vi "SLSC_Check Connection and Module.vi"(8 "error in (no error)":errorcluster, 10 "compiled.settings":T3={"Name"="", "SLSC IP -Module Name"="", "Slot #"=0, "Configuration Data"={"Properties"={"Boolean Properties"=[], "Double Properties"=[], "I32 Properties"=[], "I64 Properties"=[], "String Properties"=[], "U32 Properties"=[], "U64 Properties"=[]}}, "SLSC Set Properties"=[], "SLSC Get Properties"=[], "SLSC Commands"=[], "Username"="admin", "Password"="", "Support Modules"=[]} {"Configuration Data"."Properties"."U64 Properties"."UInt64 Write" format="%.0x"; "Configuration Data"."Properties"."U32 Properties"."UInt32 Write" format="%.0x"; "Configuration Data"."Properties"."Double Properties"."Double Write" format="%_20g"}, 11 "Item Ref in":T2 format="%.0x") -> (0 "error out":errorcluster, 1 "Device Found?":bool, 2 "compiled.settings out":T3={"Name"="", "SLSC IP -Module Name"="", "Slot #"=0, "Configuration Data"={"Properties"={"Boolean Properties"=[], "Double Properties"=[], "I32 Properties"=[], "I64 Properties"=[], "String Properties"=[], "U32 Properties"=[], "U64 Properties"=[]}}, "SLSC Set Properties"=[], "SLSC Get Properties"=[], "SLSC Commands"=[], "Username"="admin", "Password"="", "Support Modules"=[]} {"Configuration Data"."Properties"."U64 Properties"."UInt64 Write" format="%.0x"; "Configuration Data"."Properties"."U32 Properties"."UInt32 Write" format="%.0x"; "Configuration Data"."Properties"."Double Properties"."Double Write" format="%_20g"}, 3 "Item Ref out":T2 format="%.0x")   [LabVIEW 2020, in "SLSC-12201 DIO Engine.lvlib"]
uses:
  SLSC-12201 DIO Engine.lvlib
  Shared/Compiled.Settings
  Shared/SLSC Dynamic Channel.ctl
  Shared/SLSC Dynamic Channel Type.ctl
  <vilib>/NI VeriStand/Custom Device API/Custom Device Item Ref.ctl
  <vilib>/NI VeriStand/Custom Device Tools/Custom Device Utility Library/RT Debug String Color Spec.ctl
  <vilib>/SLSC/Initialize Session with Devices.vi
  <vilib>/SLSC/Close Session.vi
  <vilib>/SLSC/SLSC.lvlib
  <resource>/objmgr/slsc.rc
  <vilib>/SLSC/Initialize Session without Resources.vi
  <vilib>/NI VeriStand/Custom Device Tools/Custom Device Utility Library/Custom Device Utility Library.lvlib
  Shared/SLSC-12201 DIO Shared.lvlib
  <vilib>/NI VeriStand/Custom Device API/Custom Device API.lvlib
panel:
  out "Supported Modules":T1(array[cluster]) {"Dev.ProductNumber" format="%.0x"; "Dev.VendorNumber" format="%.0x"}
  out "Dev.VendorNum":u32 format="%.0x"
  out "Dev.ProductNum":u32 format="%.0x"
  out "Dev.ProductName":string
  in  "Connect timeout (s)":dbl=20.0 format="%#_13g"
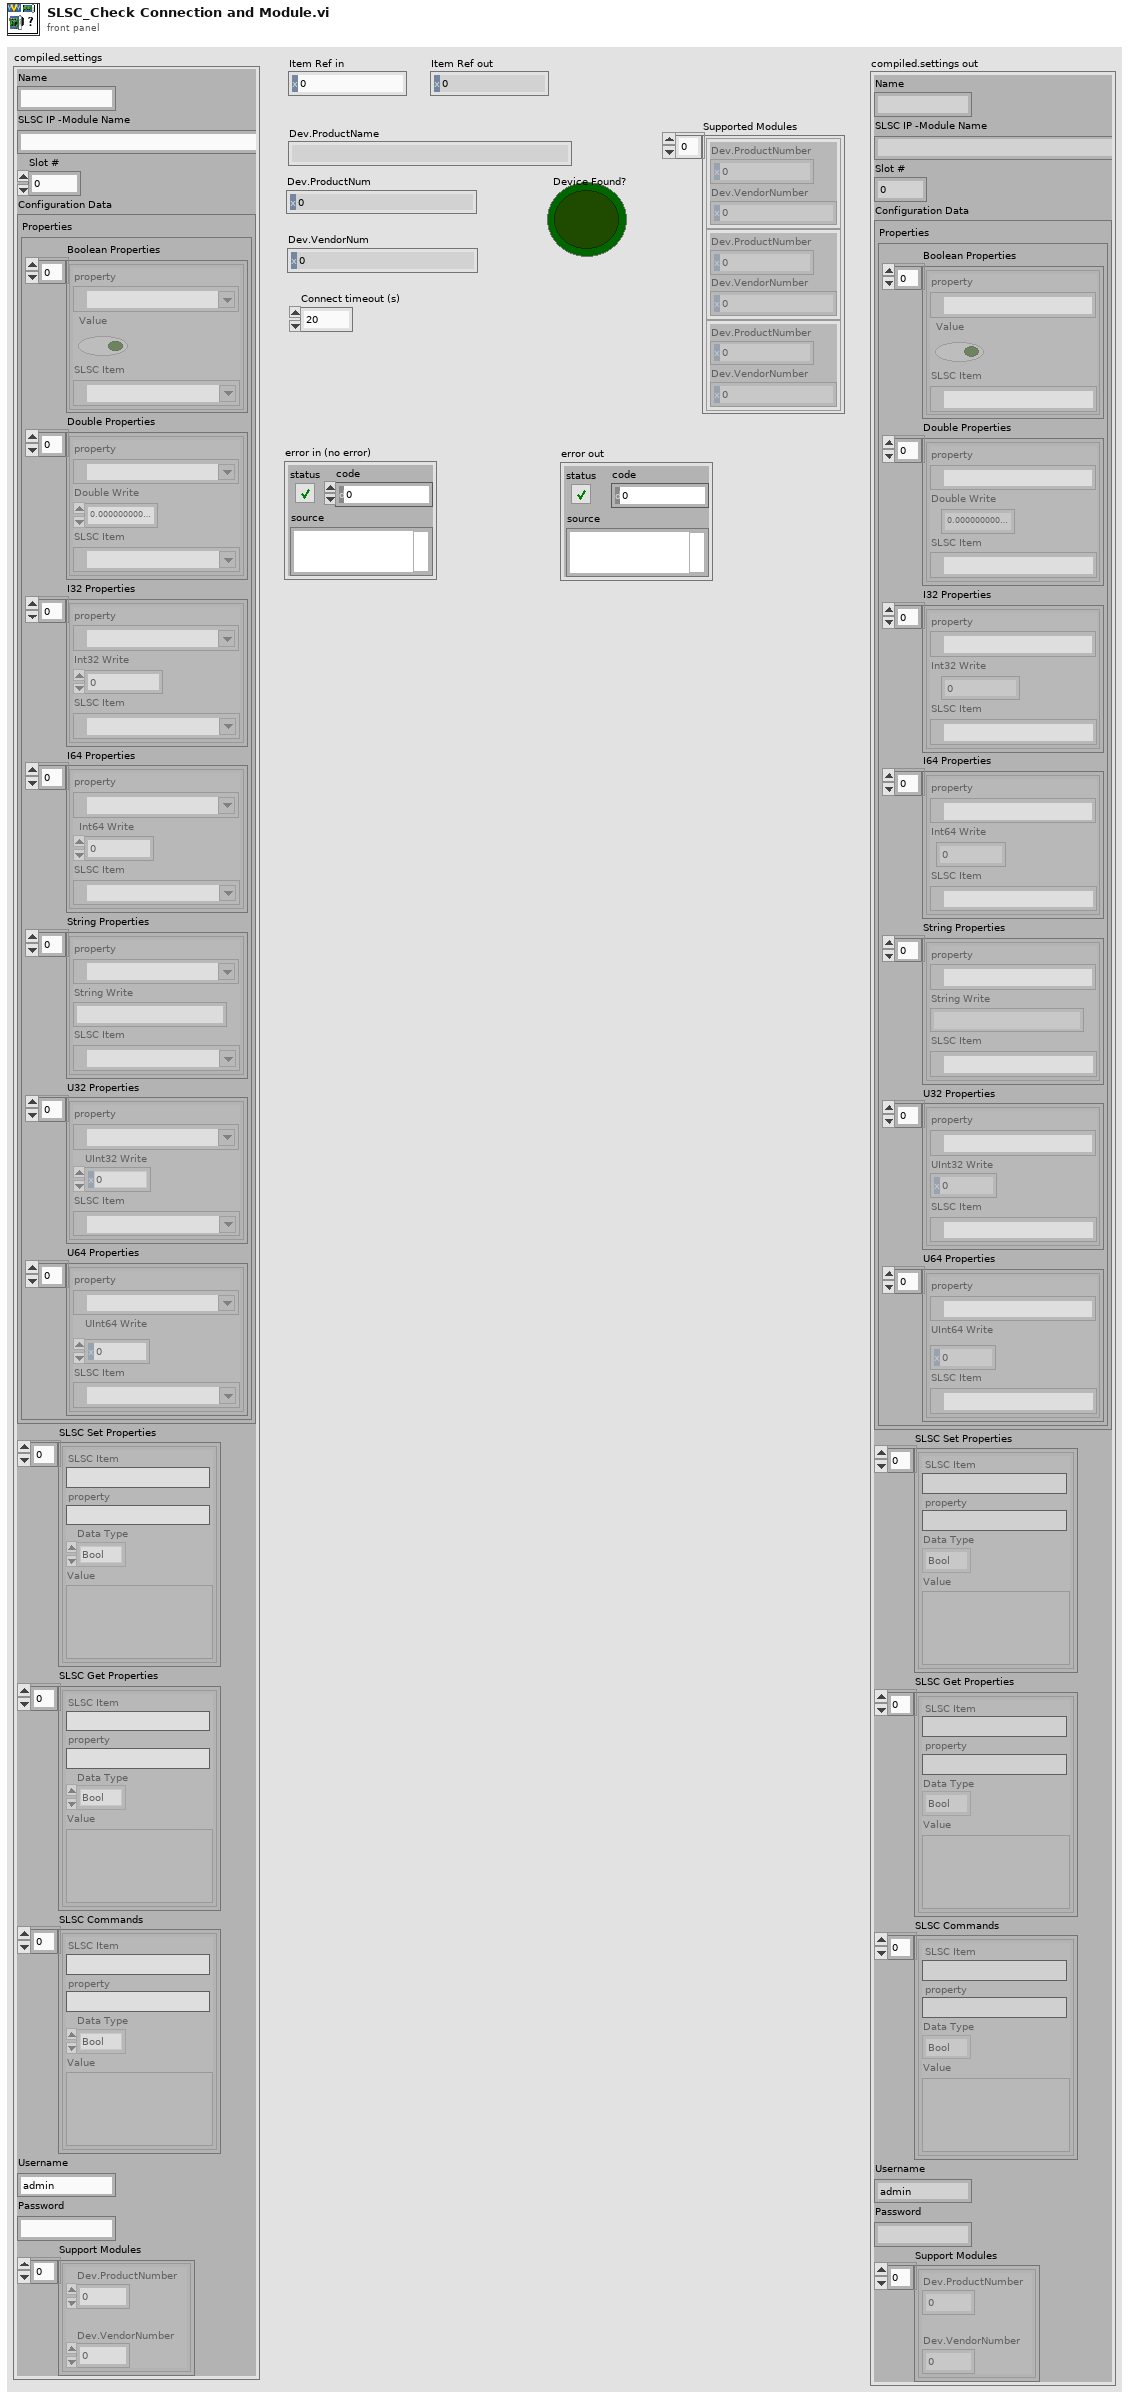
[diagram p1: front panel]
types:
  T1 = cluster{"Dev.ProductNumber":u32, "Dev.VendorNumber":u32}[]
  T2 = typedef "Custom Device API.lvlib/Custom Device Item Ref.ctl" = u64
  T3 = typedef "SLSC-12201 DIO Shared.lvlib/Compiled.Settings" = cluster{"Name":string, "SLSC IP -Module Name":string, "Slot #":i32, "Configuration Data":cluster{"Properties":cluster{"Boolean Properties":cluster{"property":refnum<k21>, "Value":bool, "SLSC Item":refnum<k21>}[], "Double Properties":cluster{"property":refnum<k21>, "Double Write":dbl, "SLSC Item":refnum<k21>}[], "I32 Properties":cluster{"property":refnum<k21>, "Int32 Write":i32, "SLSC Item":refnum<k21>}[], "I64 Properties":cluster{"property":refnum<k21>, "Int64 Write":i64, "SLSC Item":refnum<k21>}[], "String Properties":cluster{"property":refnum<k21>, "String Write":string, "SLSC Item":refnum<k21>}[], "U32 Properties":cluster{"property":refnum<k21>, "UInt32 Write":u32, "SLSC Item":refnum<k21>}[], "U64 Properties":cluster{"property":refnum<k21>, "UInt64 Write":u64, "SLSC Item":refnum<k21>}[]}}, "SLSC Set Properties":T4[], "SLSC Get Properties":T4[], "SLSC Commands":T4[], "Username":string, "Password":string, "Support Modules":cluster{"Dev.ProductNumber":u32, "Dev.VendorNumber":u32}[]}
  T4 = typedef "SLSC-12201 DIO Shared.lvlib/SLSC Dynamic Channel.ctl" = cluster{"SLSC Item":string, "property":string, "Data Type":T5, "Value":variant}
  T5 = typedef "SLSC-12201 DIO Shared.lvlib/SLSC Dynamic Channel Type.ctl" = enum16{"Bool", "Double", "I32", "I64", "String", "U32", "U64", "EnumI32"}
  T6 = typedef "Custom Device Utility Library.lvlib/RT Debug String Color Spec.ctl" = u16
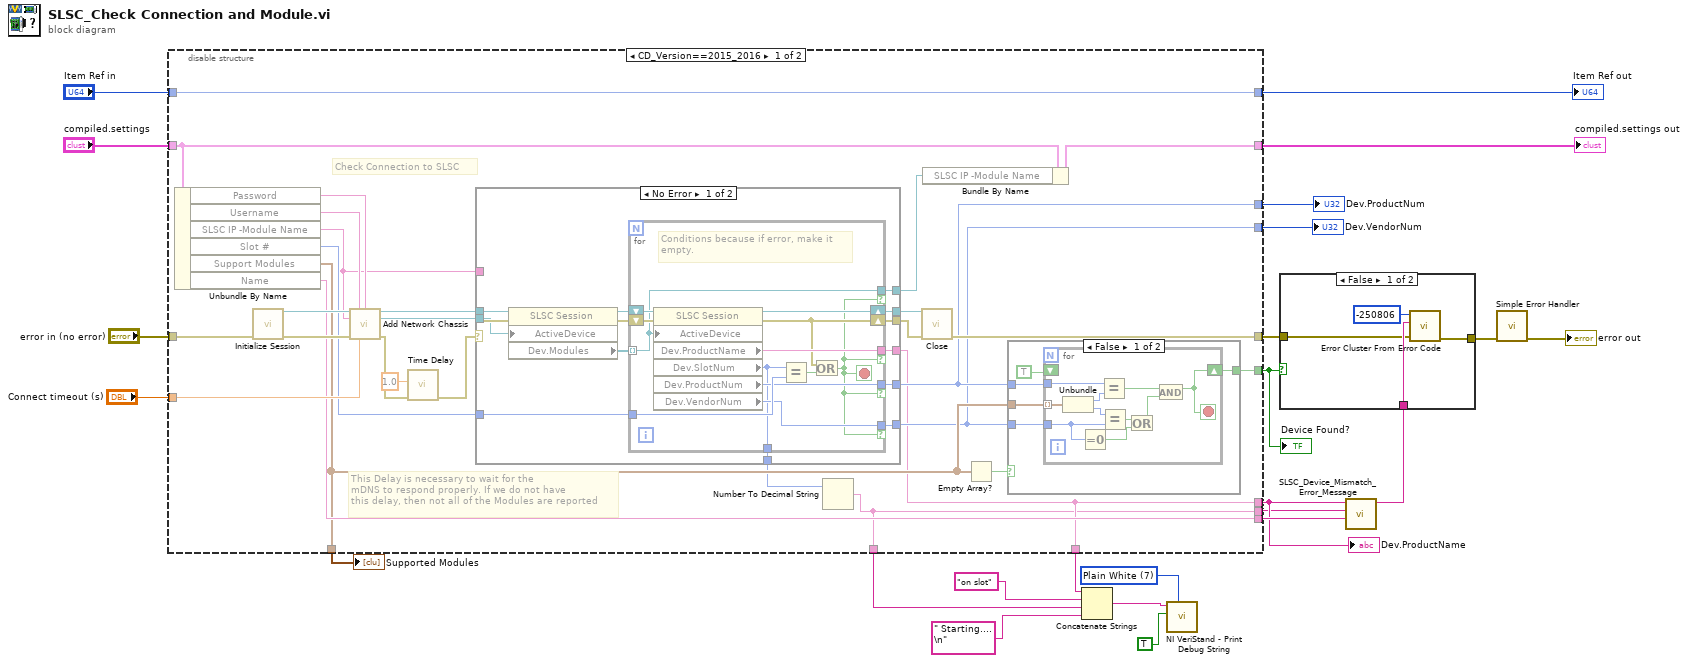
[diagram p0: block diagram]
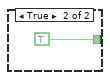
[diagram p2: hidden frame]
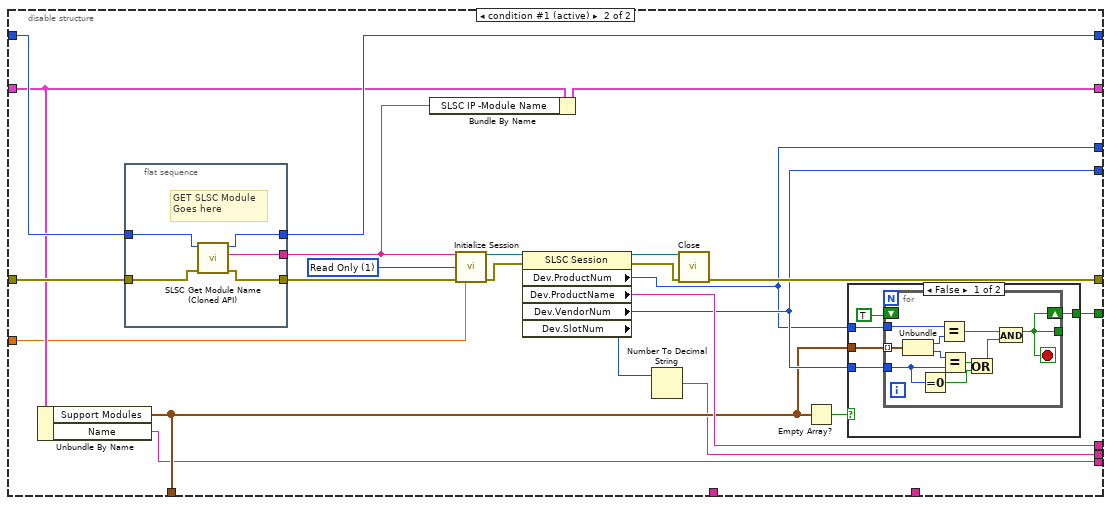
[diagram p4: hidden frame]
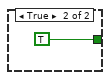
[diagram p5: hidden frame]
diagram:
  w1 = T6 7 items=["Plain White"=7, "Bold White"=15, "Bold Blue"=9, "Bold Green"=10, "Bold Red"=12] ("Attribute")
  n1 = disable-structure shown="CD_Version==2015_2016" {
    disable-tunnel: "error in (no error)" -> [w53 w119]
    disable-tunnel: "Connect timeout (s)" -> [w50 w109]
    disable-tunnel: [w43 w110] -> w22
    disable-tunnel: [w42 w101] -> w20
    disable-tunnel: [w27 w108] -> w12
    disable-tunnel: [w40 w106] -> w17
    disable-tunnel: "compiled.settings" -> [w34 w113]
    disable-tunnel: [w33 w118] -> w15
    disable-tunnel: [w41 w121] -> w14
    disable-tunnel: "Item Ref in" -> [w41 w120]
    disable-tunnel: [w38 w102] -> w11
    disable-tunnel: [w37 w103] -> w10
    disable-tunnel: [w36 w104] -> w9
    disable-tunnel: [w26 w99] -> w8
    disable-tunnel: [w27 _] -> w5
    disable-tunnel: [w26 _] -> w2
    frame condition #0 {
      # "This Delay is necessary to wait for the \nmDNS to respond properly. If we do not have\nthis delay, then not all of the Modules are reported"
      # "Check Connection to SLSC"
      n2 = Unbundle By Name(w34) -> ("Password"=w48:string, "Username"=w47:string, "SLSC IP -Module Name"=w31:string, "Slot #"=w44:i32, "Support Modules"=w38:T1, "Name"=w42:string)
      n3 = call-poly <vilib>:"Initialize Session.vi"("error in (no error)"=w53) -> ("session out"=w51:refnum<k21>, "error out"=w49:errorcluster)  [unwired: 13 in]
      n4 = call <vilib>:"Add Network Chassis.vi"("session in"=w51, "username"=w47, "password"=w48, "chassis IP address/hostname"=w31, "error in (no error)"=w49, "connect timeout (60 sec)"=w50) -> ("session out"=w52:refnum<k21>, "chassis out"=w30:refnum<k21>, "error out"=w29:errorcluster)  [unwired: 7 in]
      n5 = call "Time Delay"("error in (no error)"=w29, "Delay Time (s)"=1.0) -> ("error out"=w28:errorcluster)  [unwired: 9 in]
      n6 = case shown="No Error" w28 {
        selector: w28 -> [w76 w97]
        tunnel: w52 -> [w83 w98]
        tunnel: [w81 _] -> w27
        tunnel: [w80 w98] -> w46
        tunnel: [w79 w97] -> w45
        tunnel: w44 -> [w77 _]
        tunnel: [w75 _] -> w37
        tunnel: [w74 _] -> w36
        tunnel: [w73 _] -> w35
        tunnel: [w72 w96] -> w32
        tunnel: w31 -> [_ w96]
        tunnel: w30 -> [w70 _]
        frame No Error {
          n7 = property class="SLSC Session"(reference=w83, error in=w76, "ActiveDevice"=w70) -> (reference out=w82:refnum<k21>, error out=w78:errorcluster, "Dev.Modules"=w71:refnum<k21>[])
          n8 = for {
            tunnel: [w94] -> w81 if=w84
            shift-right: [w93] -> w80
            shift-left: w82 -> [w95]
            tunnel: w71 -> [w85] mode=indexing
            tunnel: w77 -> [w92]
            shift-right: [w89] -> w79
            shift-left: w78 -> [w90]
            tunnel: [w88] -> w75 if=w84
            tunnel: [w87] -> w74 if=w84
            tunnel: [w86] -> w73
            tunnel: [w85] -> w72 if=w84
            stop <- w84 stop-if-true
            # "Conditions because if error, make it \nempty."
            n9 = property class="SLSC Session"(reference=w95, error in=w90, "ActiveDevice"=w85) -> (reference out=w93:refnum<k21>, error out=w89:errorcluster, "Dev.ProductName"=w94:string, "Dev.SlotNum"=w86:u32, "Dev.ProductNum"=w88:u32, "Dev.VendorNum"=w87:u32)
            n10 = Equal?(x=w86, y=w92) -> (x = y?=w91:bool)
            n11 = Or(x=w89, y=w91) -> (x .or. y?=w84:bool)
          }
        }
        frame Error {
        }
      }
      n12 = Number To Decimal String(number=w35) -> (decimal integer string=w26:string)  [unwired: 1 in]
      n13 = call-poly <vilib>:"Close.vi"("session in"=w46, "error in (no error)"=w45) -> ("error out"=w43:errorcluster)  [unwired: 13 in]
      n14 = Bundle By Name(cluster=w34, "SLSC IP -Module Name"=w32) -> (w33:T3)
      n15 = Empty Array?(array=w38) -> (empty?=w39:bool)
      n16 = case shown="False" w39 {
        tunnel: w37 -> [w57 _]
        tunnel: w38 -> [w56 _]
        tunnel: w36 -> [w55 _]
        tunnel: [w54 TRUE] -> w40
        frame False {
          n17 = for {
            tunnel: w57 -> [w68]
            tunnel: w56 -> [w67] mode=indexing
            shift-right: [w63] -> w54
            shift-left: TRUE ("x = y?") -> [_]
            tunnel: w55 -> [w62]
            stop <- w63 stop-if-true
            n18 = Unbundle(w67) -> ("Dev.ProductNumber"=w65:u32, "Dev.VendorNumber"=w64:u32)
            n19 = Equal To 0?(x=w62) -> (x = 0?=w60:bool)
            n20 = Equal?(x=w68, y=w65) -> (x = y?=w66:bool)
            n21 = Equal?(x=w64, y=w62) -> (x = y?=w61:bool)
            n22 = Or(x=w61, y=w60) -> (x .or. y?=w59:bool)
            n23 = And(x=w66, y=w59) -> (x .and. y?=w63:bool)
          }
        }
        frame True {
        }
      }
    }
    frame condition #1 (active) {
      w105 = 1 items=["None"=0, "Read Only"=1, "Read/Write"=3] ("reservation access (Read/Write)")
      n24 = Unbundle By Name(w113) -> ("Support Modules"=w102:T1, "Name"=w101:string)
      n25 = flat-sequence {
        tunnel: [w140] -> w121
        tunnel: w120 -> [w141]
        tunnel: [w138] -> w116
        tunnel: w119 -> [w139]
        tunnel: [w142] -> w117
        frame #0 {
          # "GET SLSC Module\nGoes here"
          n26 = call "SLSC Get Module Name (Cloned API).vi"("error in (no error)"=w139, "Item Ref in"=w141) -> ("error out"=w138:errorcluster, "SLSC Module"=w142:string, "Item Ref out"=w140:T2)  [unwired: 7 in]
        }
      }
      n27 = Bundle By Name(cluster=w113, "SLSC IP -Module Name"=w117) -> (w118:T3)
      n28 = call-poly <vilib>:"Initialize Session.vi"("devices"=w117, "reservation access (Read/Write)"=w105, "error in (no error)"=w116, "connect timeout (60 sec)"=w109) -> ("session out"=w115:refnum<k21>, "error out"=w114:errorcluster)  [unwired: 10 in]
      n29 = property class="SLSC Session"(reference=w115, error in=w114) -> (reference out=w112:refnum<k21>, error out=w111:errorcluster, "Dev.ProductNum"=w103:u32, "Dev.ProductName"=w108:string, "Dev.VendorNum"=w104:u32, "Dev.SlotNum"=w100:u32)
      n30 = Number To Decimal String(number=w100) -> (decimal integer string=w99:string)  [unwired: 1 in]
      n31 = call-poly <vilib>:"Close.vi"("session in"=w112, "error in (no error)"=w111) -> ("error out"=w110:errorcluster)  [unwired: 13 in]
      n32 = Empty Array?(array=w102) -> (empty?=w107:bool)
      n33 = case shown="False" w107 {
        tunnel: w103 -> [w125 _]
        tunnel: w102 -> [w124 _]
        tunnel: w104 -> [w123 _]
        tunnel: [w122 TRUE] -> w106
        frame False {
          n34 = for {
            tunnel: w125 -> [w136]
            tunnel: w124 -> [w135] mode=indexing
            tunnel: [w131] -> _
            shift-right: [w131] -> w122
            shift-left: TRUE ("x = y?") -> [_]
            tunnel: w123 -> [w130]
            stop <- w131 stop-if-true
            n35 = Unbundle(w135) -> ("Dev.ProductNumber"=w133:u32, "Dev.VendorNumber"=w132:u32)
            n36 = Equal To 0?(x=w130) -> (x = 0?=w128:bool)
            n37 = Equal?(x=w136, y=w133) -> (x = y?=w134:bool)
            n38 = Equal?(x=w132, y=w130) -> (x = y?=w129:bool)
            n39 = Or(x=w129, y=w128) -> (x .or. y?=w127:bool)
            n40 = And(x=w134, y=w127) -> (x .and. y?=w131:bool)
          }
        }
        frame True {
        }
      }
    }
  }
  "Dev.ProductName" <- w12
  "compiled.settings out" <- w15
  "Item Ref out" <- w14
  "Device Found?" <- w17
  "Supported Modules" <- w11
  "Dev.ProductNum" <- w10
  "Dev.VendorNum" <- w9
  n41 = Concatenate Strings(w5, "on slot" ("Message"), w2, " Starting....\n" ("Message")) -> (w6:string)
  n42 = call <vilib>:"NI VeriStand - Print Debug String.vi"("Attribute"=w1, "Add to log file? (F)"=TRUE ("Add to log file? (T)"), "Message"=w6) -> ()  [unwired: 8 in, 1 out]
  n43 = call "SLSC_Device_Mismatch_Error_Message.vi"("Name"=w20, "Slot Number"=w8, "Product Name"=w12) -> ("String"=w21:string)  [unwired: 8 in]
  n44 = case shown="False" w17 {
    tunnel: [w146 w147] -> w19
    tunnel: w22 -> [w143 w147]
    tunnel: w21 -> [w144 _]
    frame False {
      n45 = call <vilib>:"Error Cluster From Error Code.vi"("error in (no error)"=w143, "error message (\"\")"=w144, "error code (0)"=-250806) -> ("error out"=w146:errorcluster)  [unwired: 6 in]
    }
    frame True {
    }
  }
  n46 = call <vilib>:"Simple Error Handler.vi"("error in (no error)"=w19) -> ("error out"=→"error out":errorcluster)  [unwired: 4 in, 4 out]
